vi "Init.vi"(8 "error in (no error)":errorcluster, 11 "UI Actor in":refnum<class "UI Actor.lvclass">) -> (0 "error out":errorcluster, 3 "UI Actor out":refnum<class "UI Actor.lvclass">)   [LabVIEW 2020, in "UI Actor.lvlib" / "UI Actor.lvclass"]
uses:
  UI Actor.lvclass
  C:/Program Files/National Instruments/LabVIEW 2020/vi.lib/ActorFramework/Actor/Actor.lvclass
  Msg/Msg.lvclass
  UI Actor.lvclass/UI Actor.ctl
  Coffee Actor/Coffee Actor.lvclass
  Coffee Actor/Coffee Actor.lvclass/Coffee Actor.ctl
  Soda Actors/Soda Actors.lvclass
  Soda Actors/Soda Actors.lvclass/Soda Actors.ctl
  MXN Actor/MXN Actor.lvclass
  MXN Actor/MXN Actor.lvclass/MXN Actor.ctl
  USD Actor/USD Actor.lvclass
  USD Actor/USD Actor.lvclass/USD Actor.ctl
  Msg/Msg.lvclass/Msg.ctl
  Get Coins.vi
  Get Sub Panel Coins.vi
  Get Products.vi
  Get Sub Panel Prods.vi
  Get Sub Panel Msg.vi
  <vilib>/ActorFramework/Actor/Actor.lvclass
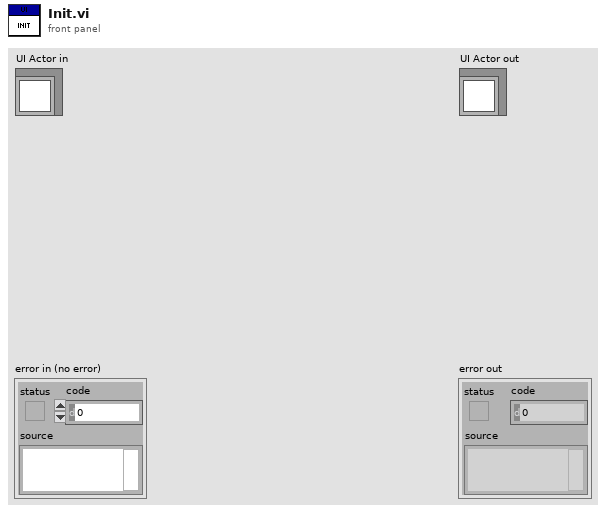
[diagram p1: front panel]
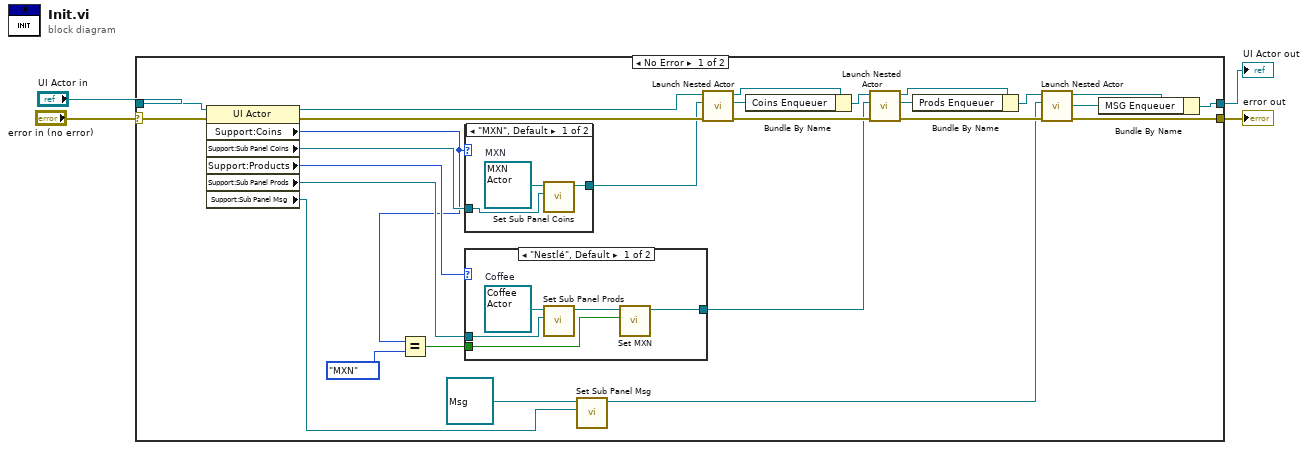
[diagram p0: block diagram]
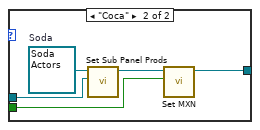
[diagram p2: hidden frame]
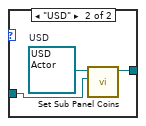
[diagram p3: hidden frame]
diagram:
  n1 = case shown="No Error" "error in (no error)" {
    selector: "error in (no error)" -> [w31 w49]
    tunnel: [w15 w49] -> w3
    tunnel: [w12 w48] -> w1
    tunnel: "UI Actor in" -> [w30 w48]
    frame No Error {
      n2 = property class="UI Actor"(reference=w30, error in=w31) -> (reference out=w20:refnum<class "UI Actor.lvclass">, error out=w22:errorcluster, "Support:Coins"=w7:enum16{"MXN", "USD"}, "Support:Sub Panel Coins"=w26:refnum<vi>, "Support:Products"=w25:enum16{"Nestlé", "Coca"}, "Support:Sub Panel Prods"=w24:refnum<vi>, "Support:Sub Panel Msg"=w9:refnum<vi>)
      n3 = Equal?(x=w7, y=enum16{"MXN", "USD"}."MXN") -> (x = y?=w5:bool)
      n4 = case shown="\"MXN\", Default" w7 {
        tunnel: [w43 w46] -> w17
        tunnel: w26 -> [w42 w45]
        frame "MXN", Default {
          w44 = refnum<class "MXN Actor.lvclass"> refnum  # MXN
          n5 = call "Set Sub Panel Coins.vi"("Sub Panel Coins"=w42, "MXN Actor in"=w44) -> ("MXN Actor out"=w43:refnum<class "MXN Actor.lvclass">)  [unwired: 8 in, 1 out]
        }
        frame "USD" {
          w47 = refnum<class "USD Actor.lvclass"> refnum  # USD
          n6 = call "Set Sub Panel Coins.vi"("Sub Panel Coins"=w45, "USD Actor in"=w47) -> ("USD Actor out"=w46:refnum<class "USD Actor.lvclass">)  [unwired: 8 in, 1 out]
        }
      }
      n7 = case shown="\"Nestlé\", Default" w25 {
        tunnel: w24 -> [w35 w40]
        tunnel: [w33 w38] -> w16
        tunnel: w5 -> [w32 w37]
        frame "Nestlé", Default {
          w36 = refnum<class "Coffee Actor.lvclass"> refnum  # Coffee
          n8 = call "Set Sub Panel Prods.vi"("Sub Panel Prods"=w35, "Coffee Actor in"=w36) -> ("Coffee Actor out"=w34:refnum<class "Coffee Actor.lvclass">)  [unwired: 8 in, 1 out]
          n9 = call "Set MXN.vi"("MXN"=w32, "Coffee Actor in"=w34) -> ("Coffee Actor out"=w33:refnum<class "Coffee Actor.lvclass">)  [unwired: 8 in, 1 out]
        }
        frame "Coca" {
          w41 = refnum<class "Soda Actors.lvclass"> refnum  # Soda
          n10 = call "Set Sub Panel Prods.vi"("Sub Panel Prods"=w40, "Soda Actors in"=w41) -> ("Soda Actors out"=w39:refnum<class "Soda Actors.lvclass">)  [unwired: 8 in, 1 out]
          n11 = call "Set MXN.vi"("MXN"=w37, "Soda Actors in"=w39) -> ("Soda Actors out"=w38:refnum<class "Soda Actors.lvclass">)  [unwired: 8 in, 1 out]
        }
      }
      n12 = call "Set Sub Panel Msg.vi"("Sub Panel Msg"=w9, "Msg in"=refnum<class "Msg.lvclass"> refnum ("Msg.lvlib:Msg.lvclass")) -> ("Msg out"=w8:refnum<class "Msg.lvclass">)  [unwired: 8 in, 1 out]
      n13 = call <vilib>:"Launch Nested Actor.vi"("error in (no error)"=w22, "Nested Actor"=w17, "Caller Actor in"=w20) -> ("error out"=w23:errorcluster, "Nested Actor's Enqueuer"=w18:refnum<class "Message Enqueuer.lvclass">, "Caller Actor out"=w21:refnum<class "UI Actor.lvclass">)  [unwired: 6 in]
      n14 = Bundle By Name(cluster=w21, "Coins Enqueuer"=w18) -> (w19:refnum<class "UI Actor.lvclass">)
      n15 = call <vilib>:"Launch Nested Actor.vi"("error in (no error)"=w23, "Nested Actor"=w16, "Caller Actor in"=w19) -> ("error out"=w29:errorcluster, "Nested Actor's Enqueuer"=w27:refnum<class "Message Enqueuer.lvclass">, "Caller Actor out"=w28:refnum<class "UI Actor.lvclass">)  [unwired: 6 in]
      n16 = Bundle By Name(cluster=w28, "Prods Enqueuer"=w27) -> (w14:refnum<class "UI Actor.lvclass">)
      n17 = call <vilib>:"Launch Nested Actor.vi"("error in (no error)"=w29, "Nested Actor"=w8, "Caller Actor in"=w14) -> ("error out"=w15:errorcluster, "Nested Actor's Enqueuer"=w11:refnum<class "Message Enqueuer.lvclass">, "Caller Actor out"=w13:refnum<class "UI Actor.lvclass">)  [unwired: 6 in]
      n18 = Bundle By Name(cluster=w13, "MSG Enqueuer"=w11) -> (w12:refnum<class "UI Actor.lvclass">)
    }
    frame Error {
    }
  }
  "error out" <- w3
  "UI Actor out" <- w1
